vi "Create projectr.vi"(11 "error in (no error)":errorcluster) -> (4 "Comment out":string, 6 "Job & Site out":T2, 8 "Tool out":T1, 10 "OK":bool, 15 "error out":errorcluster)   [LabVIEW 2011]
doc: "Welcome screen, with basic options"
uses:
  GUI/Job setup/Job and site cluster.ctl
  emi cndiates/List of all contrys(combo box).ctl
  GUI/Job setup/Tool registration ID.ctl
  Project in icluster.ctl
  Run Information.ctl
panel:
  in  "Comment":string
  in  "Tool":T1
  in  "Job & Site":T2
  in  "Cancel":bool
  in  "OK btn":bool
  # "Comment"
  # "Tab header s can be changed as wanted\n\nCustom can be used for completly ccutom behavior,\nmust then highjack  an other hidden page, for settings"
  # "Add custom behavior taht cvan not be replicated by a simple cluster with valisdity checking"
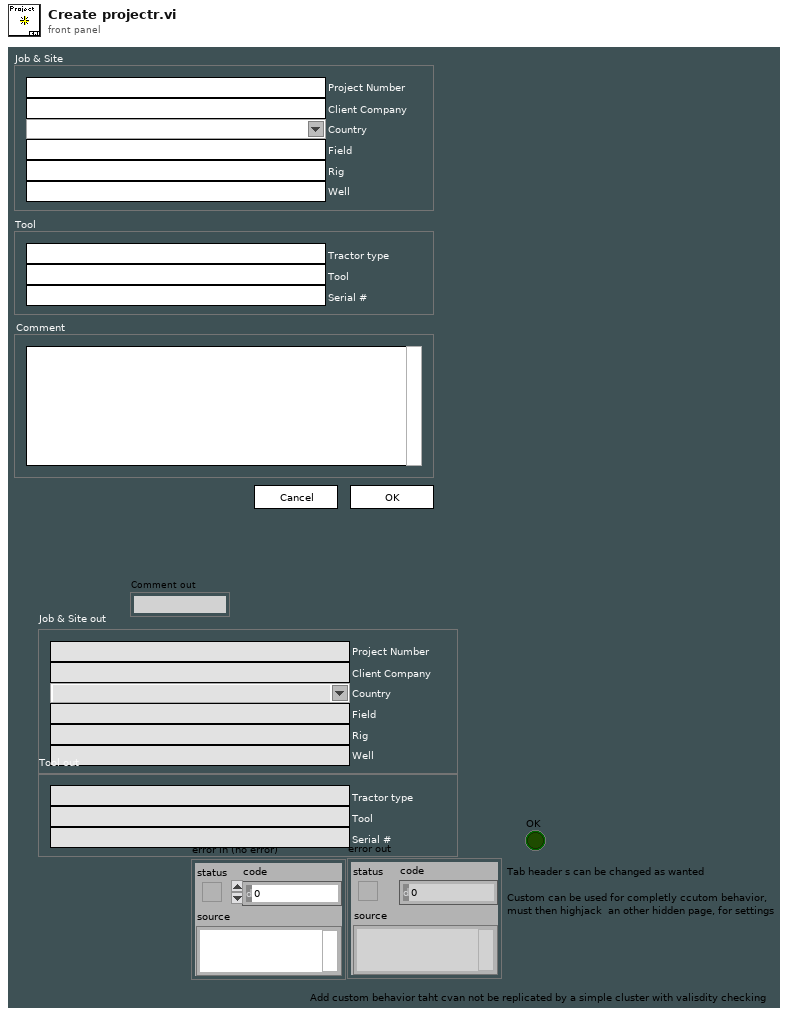
[diagram p1: front panel]
types:
  T1 = typedef "Tool registration ID.ctl" = cluster{"Tractor type":string, "Tool":string, "Serial #":string}
  T2 = typedef "Job and site cluster.ctl" = cluster{"Project Number":string, "Client Company":string, "Country":T3, "Field":string, "Rig":string, "Well":string}
  T3 = typedef "List of all contrys(combo box).ctl" = string
  T4 = typedef "Options  All pages and custom.ctl" = cluster{"P 1 (App)":T5, "P 2":T6, "P 3":T7, "P 4":T10, "P 5":T15, "P 6 (Err)":T16, "P 7 (Expert)":T17, "P 8 (Depth)":T19, "C 1":T20, "C 2":T21}
  T5 = typedef "Options Page 1 (App).ctl" = cluster{"Result files":path, "PCP Interface":string, "Tractor/Stroker Interface":string, "Tractor Interface":string, "Modem Status Interface":string, "Audible Alarm":bool, "Force alarm on Technical":bool, "Force alarm on HH":bool, "Force alarm on LL":bool, "Force alarm on H":bool, "Force alarm on L":bool}
  T6 = typedef "Options Page 2.ctl" = cluster{"Solenoid & Relay latching time":u16, "Tractor relay 1":dbl, "Tractor relay 2":dbl, "Tractor Solenoid limit":dbl}
  T7 = typedef "Options Page 3.ctl" = cluster{"Min resistance":dbl, "Max resistance":dbl, "Head voltage range":T8, "Max voltage jump":dbl, "Maximum resistance change":dbl, "Start Telemetry Voltage":dbl, "Start Telemetry Timeout":dbl, "Start Motor Voltage":dbl, "Stop Motor Voltage":dbl, "Pass Mode Warning Voltage":dbl, "Relay Switch Voltage":dbl, "Relay Status Loss Voltage":dbl, "Samples to average":i32, "PSU type DO NOT USE":T9, "Magna OVP":dbl, "Magna Current Limit":dbl}
  T8 = typedef "PCP type List.ctl" = enum16{"0 - 350V", "0 - 450V", "0 - 600V"}
  T9 = typedef "PSU Type.ctl" = enum16{"Unipower", "Magna 8.3A", "Magna 12A", "None"}
  T10 = typedef "Options Page 4.ctl" = cluster{"Solenoid & Relay latching time":u16, "Stroker relay 1":dbl, "Stroker Relay 2":dbl, "Stroker Solenoid limit":dbl, "Force det.":T11, "Stroke force lim.":dbl, "Anchor Enabled Pressure":dbl, "Tacometer puls":dbl, "Default anchor behavior":T12, "Default stroker behavior":T13, "Default stroker force limit (tonne)":dbl, "Slips Size":T14}
  T11 = typedef "Stroke force selector.ctl" = enum16{"Stroke in = node 1", "Strok out = node 1"}
  T12 = typedef "Default anchor behavior.ctl" = enum16{"Do nothing", "Set Anchor", "Release Anchor"}
  T13 = typedef "Default stroker behavior.ctl" = enum16{"Do nothing", "Stop", "Go Out", "Go In"}
  T14 = typedef "Slips Type Radio.ctl" = enum32{"No Selection", "338 MRS", "3,9 MRS"}
  T15 = typedef "Options Page 5.ctl" = cluster{"Solenoid & Relay latching time":u16, "Driller relay 1":dbl, "Driller Relay 2":dbl, "Driller  Solenoid limit":dbl}
  T16 = typedef "Options Page 6 (Err).ctl" = cluster{"Error and event files":path}
  T17 = typedef "Options Page 7 (Expert).ctl" = cluster{"Show Debug":bool, "Log debug messages":bool, "Additional debug messages":bool, "Start Beagle with Simulator data":bool, "Workshop mode":bool, "Modem baud":u16, "enumCANCOM":bool, "Modem sim":T18, "Telemetry Timeout Disable":i32, "Buffer size":i32, "Upd regular data":bool, "Cable comp":cluster{"VMOD1 Voltage(V)":dbl, "VMOD2 Voltage(V)":dbl}}
  T18 = typedef "Modem simulation setup.ctl" = cluster{"Modem dealay sim":bool, "Sim baud Tx":u16, "Bit Error fraction Tx":dbl, "Sim baud Rx":u16, "Bit Error fraction Rx":dbl}
  T19 = typedef "Options Page 8 (Depth).ctl" = cluster{"Winch Spool Circumference":dbl, "Winch Pulses per Revolution":dbl, "Current Depth":dbl}
  T20 = typedef "Options Custom 1.ctl" = cluster{"Depth Updated":bool, "Depth Offset":dbl}
  T21 = typedef "Options Custom 2.ctl" = cluster{"Placeholder":bool}
  T22 = typedef "Project in icluster.ctl" = cluster{"Job and Site":T2, "Tool":T1, "Run Information":T23}
  T23 = typedef "Run Information.ctl" = cluster{"Active Run":bool, "String Check Rec":bool, "Run Number":i32, "Time of File Start":string}
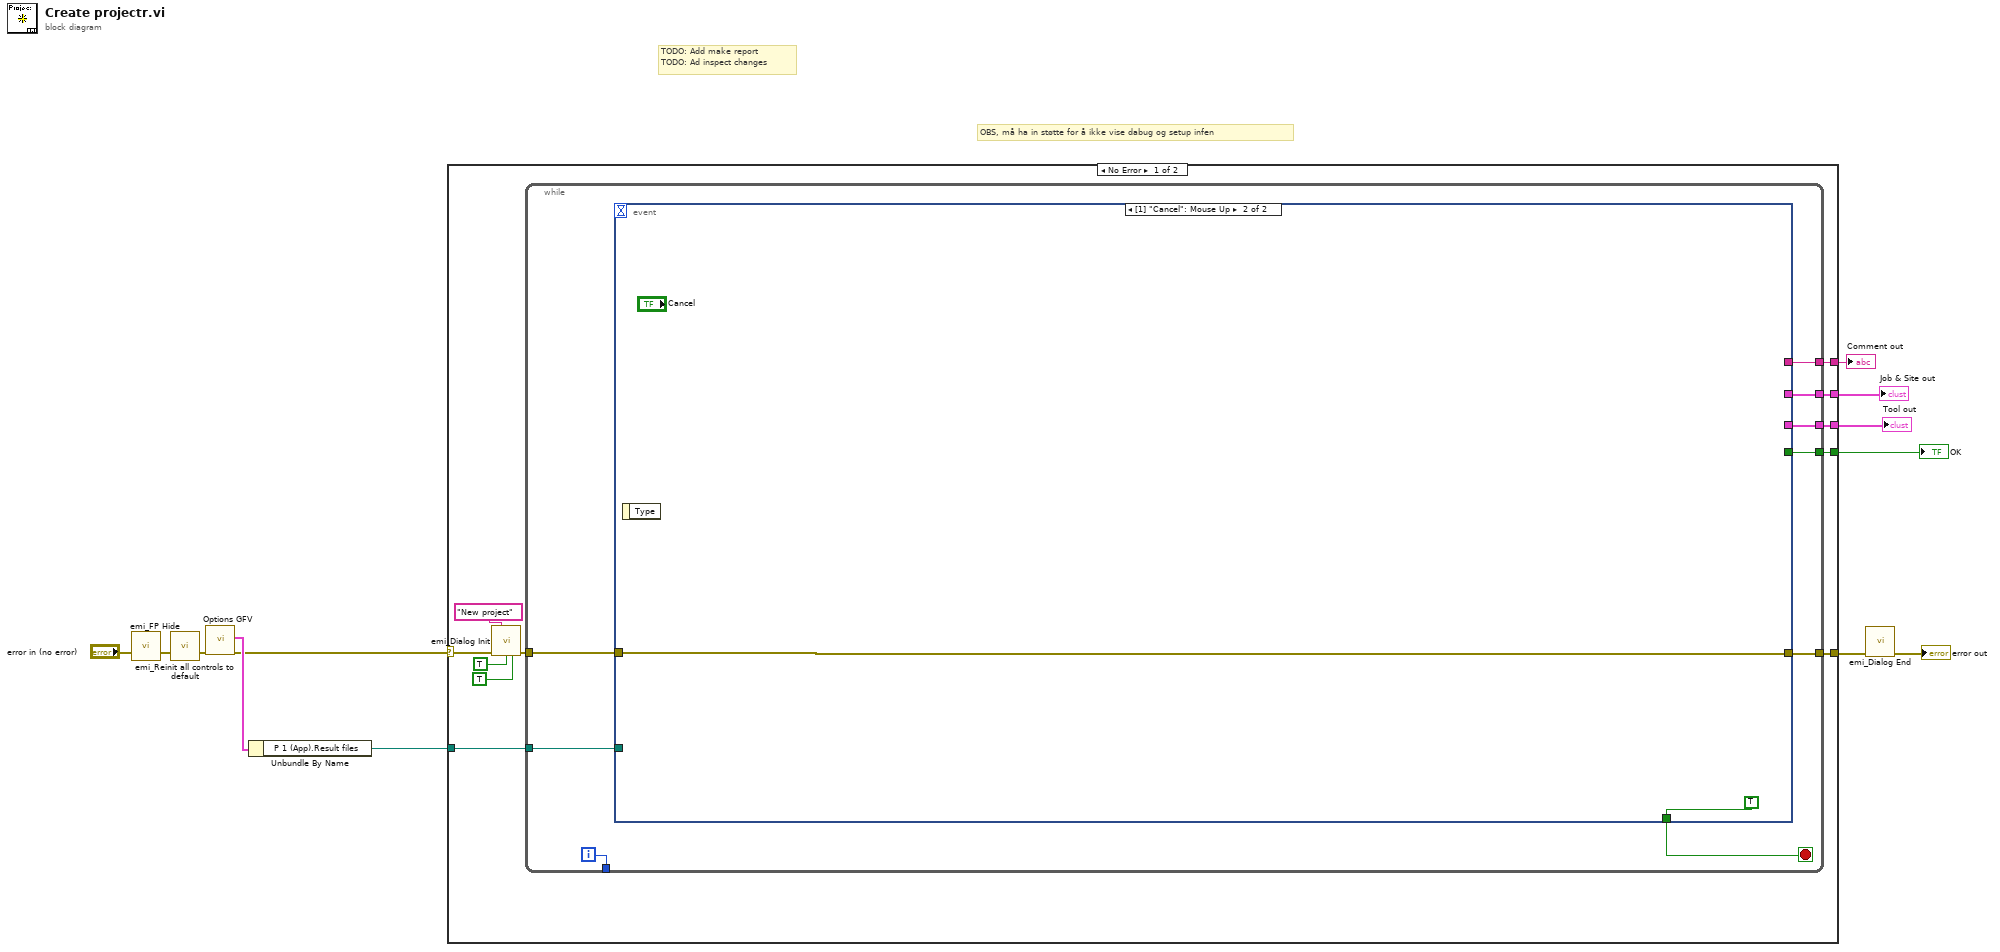
[diagram p0: block diagram]
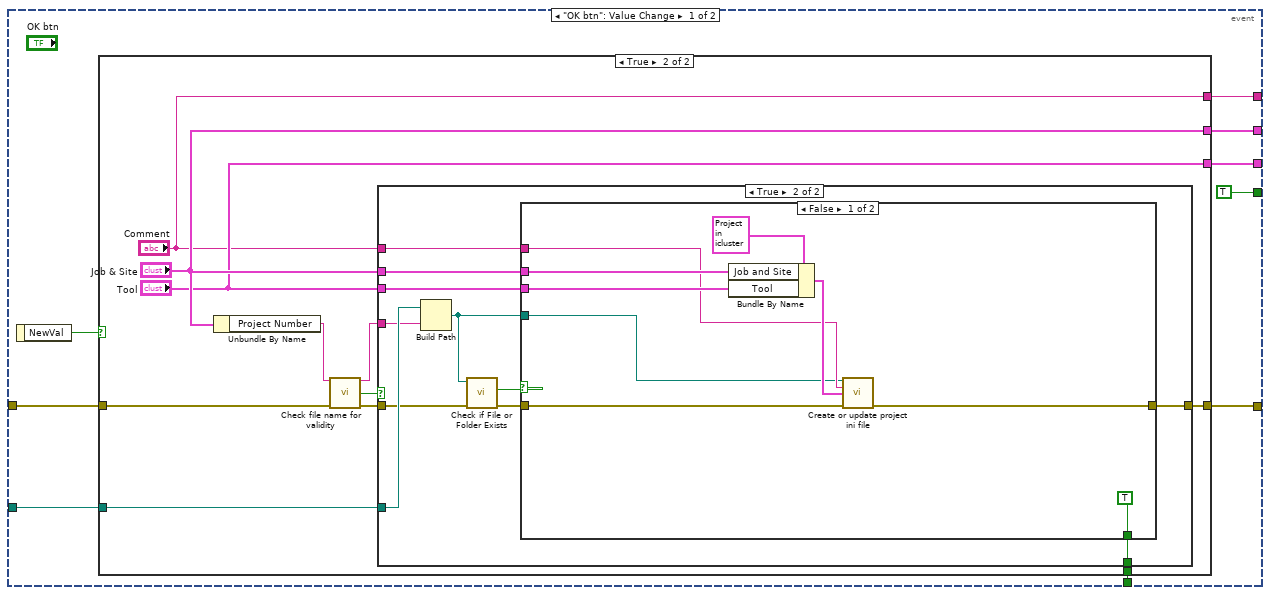
[diagram p2: hidden frame]
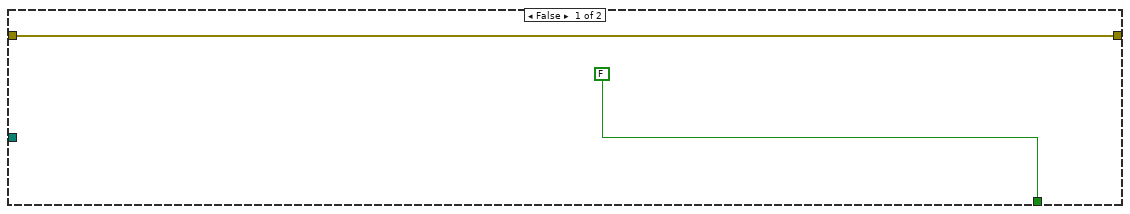
[diagram p3: hidden frame]
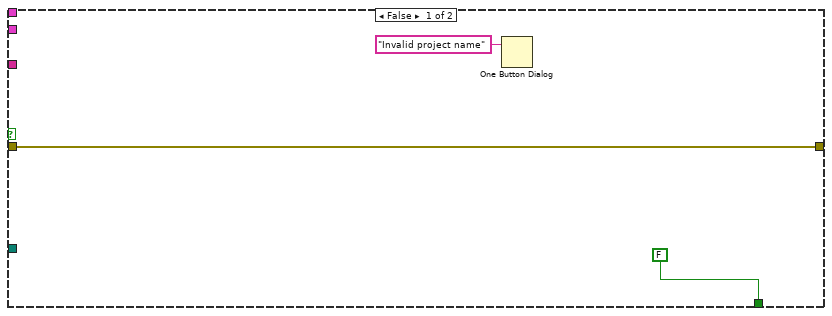
[diagram p4: hidden frame]
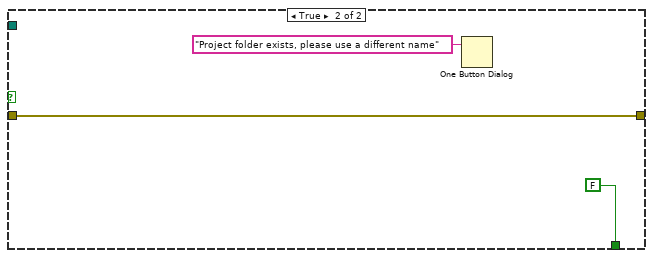
[diagram p5: hidden frame]
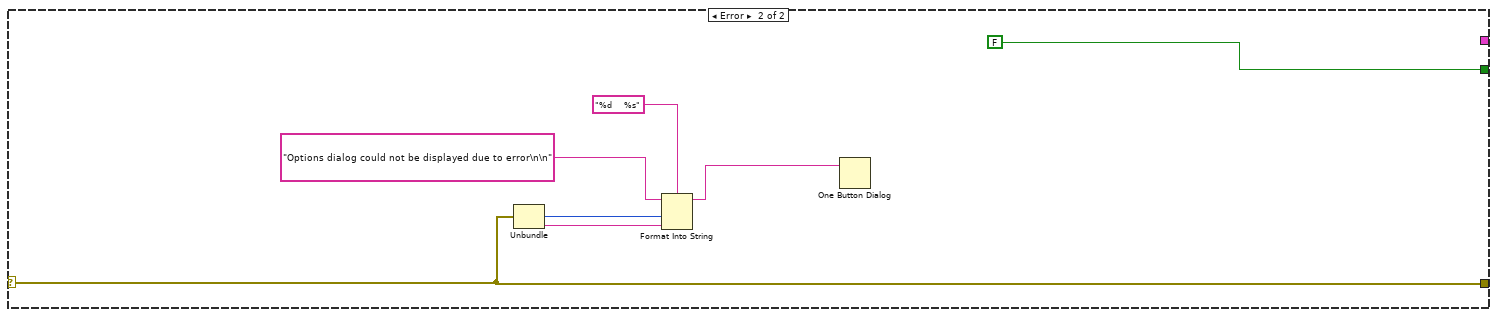
[diagram p6: hidden frame]
diagram:
  # "OBS, må ha in støtte for å ikke vise dabug og setup infen"
  # "TODO: Add make report\nTODO: Ad inspect changes"
  n1 = call "emi_FP Hide.vi"("error in (no error)"="error in (no error)") -> ("error out"=w8:errorcluster)  [unwired: 13 in, 1 out]
  n2 = call "emi_Reinit all controls to default.vi"("error in (no error)"=w8) -> ("error out"=w6:errorcluster)  [unwired: 13 in, 1 out]
  n3 = call "Options GFV.vi"("error in (no error)"=w6) -> ("Options"=w7:T4, "error out"=w5:errorcluster)  [unwired: 16 in, 1 out]
  n4 = Unbundle By Name(w7) -> ("P 1 (App).Result files"=w4:path)
  n5 = case shown="No Error" w5 {
    selector: w5 -> [w18 w88]
    tunnel: [w23 FALSE] -> w11
    tunnel: [w22 w88] -> w10
    tunnel: w4 -> [w16 _]
    tunnel: [w15 _] -> w3
    tunnel: [w14 _] -> w2
    tunnel: [w13 _] -> w1
    frame No Error {
      n6 = call "emi_Dialog Init.vi"("Header String(\"\")"="New project" ("Header String(\"\")"), "error in"=w18, "Set BG Color(T)"=TRUE, "Modal(T)"=TRUE) -> ("error out"=w21:errorcluster)  [unwired: 11 in]
      n7 = while {
        tunnel: [w32] -> _
        tunnel: w21 -> [w30]
        tunnel: [w29] -> w22
        tunnel: [w28] -> w23
        tunnel: w16 -> [w27]
        tunnel: [w26] -> w15
        tunnel: [w25] -> w14
        tunnel: [w24] -> w13
        i -> [w32]
        stop <- w31 stop-if-true
        n8 = event shown="[1] \"Cancel\": Mouse Up" {
          selector: _ -> [_ _]
          dyn-events: _ -> [_ _]
          timeout: _ -> [_ _]
          tunnel: [w39 TRUE] -> w31
          tunnel: w30 -> [w35 w81]
          tunnel: [w38 w81] -> w29
          tunnel: [TRUE _] -> w28
          tunnel: w27 -> [w40 _]
          tunnel: [w37 _] -> w26
          tunnel: [w36 _] -> w25
          tunnel: [w33 _] -> w24
          event "OK btn": Value Change {
            n9 = event-data() -> ("NewVal"=w34:bool)  [unwired: 1 in]
            n10 = case shown="True" w34 {
              tunnel: w40 -> [_ w54]
              tunnel: [FALSE w53] -> w39
              tunnel: [w42 w52] -> w38
              tunnel: [_ "Job & Site"] -> w37
              tunnel: [_ "Tool"] -> w36
              tunnel: w35 -> [w42 w49]
              tunnel: [_ "Comment"] -> w33
              frame False {
              }
              frame True {
                n11 = Unbundle By Name("Job & Site") -> ("Project Number"=w46:string)
                n12 = call "Check file name for validity.vi"("String in"=w46, "error in (no error)"=w49) -> ("String out"=w45:string, "Valid File of folder name"=w47:bool, "error out"=w48:errorcluster)  [unwired: 11 in]
                n13 = case shown="True" w47 {
                  tunnel: w54 -> [_ w68]
                  tunnel: [FALSE w67] -> w53
                  tunnel: [w57 w64] -> w52
                  tunnel: "Job & Site" -> [_ w62]
                  tunnel: "Tool" -> [_ w61]
                  tunnel: w48 -> [w57 w60]
                  tunnel: w45 -> [_ w59]
                  tunnel: "Comment" -> [_ w58]
                  frame False {
                    n14 = One Button Dialog(message="Invalid project name") -> ()  [unwired: 1 in, 1 out]
                  }
                  frame True {
                    n15 = Build Path(base path=w68, name or relative path=w59) -> (appended path=w63:path)
                    n16 = call <vilib>:"Check if File or Folder Exists.vi"("error in (no error)"=w60, "path"=w63) -> ("error out"=w65:errorcluster, "file or folder exists?"=w66:bool)  [unwired: 7 in, 1 out]
                    n17 = case shown="False" w66 {
                      tunnel: [TRUE FALSE] -> w67
                      tunnel: w65 -> [w70 w78]
                      tunnel: [w72 w78] -> w64
                      tunnel: w63 -> [w69 _]
                      tunnel: w61 -> [w74 _]
                      tunnel: w62 -> [w73 _]
                      tunnel: w58 -> [w71 _]
                      frame False {
                        n18 = Bundle By Name(cluster=T22 {"Job and Site"={"Project Number"="test", "Client Company"="test", "Country"="test", "Field"="test", "Rig"="Afghanistan", "Well"=""}, "Tool"={"Tractor type"="test", "Tool"="test", "Serial #"="test"}, "Run Information"={"Active Run"=FALSE, "String Check Rec"=FALSE, "Run Number"=0, "Time of File Start"=""}} ("Project information"), "Job and Site"=w73, "Tool"=w74) -> (w75:T22)
                        n19 = call "Create or update project ini file.vi"("Project file path"=w69, "Comment"=w71, "Project information"=w75, "error in (no error)"=w70) -> ("error out"=w72:errorcluster)  [unwired: 11 in]
                      }
                      frame True {
                        n20 = One Button Dialog(message="Project folder exists, please use a different name") -> ()  [unwired: 1 in, 1 out]
                      }
                    }
                  }
                }
              }
            }
          }
          event "Cancel": Mouse Up {
            n21 = event-data() -> ()  [unwired: 1 in, 1 out]
          }
        }
      }
    }
    frame Error {
      n22 = Unbundle(w88) -> ("code"=w85:i32, "source"=w84:string)  [unwired: 1 out]
      n23 = Format Into String(format string="%d    %s", initial string="Options dialog could not be displayed due to error\n\n" ("message"), w85, w84) -> (resulting string=w86:string)  [unwired: 1 in, 1 out]
      n24 = One Button Dialog(message=w86) -> ()  [unwired: 1 in, 1 out]
    }
  }
  "OK" <- w11
  "Job & Site out" <- w3
  "Tool out" <- w2
  "Comment out" <- w1
  n25 = call "emi_Dialog End.vi"("error in"=w10) -> ("error out"=→"error out":errorcluster)  [unwired: 14 in]
